vi "Sensor Loop.vi"() -> ()   [LabVIEW 2017]
uses:
  Typedef/FGVAction.ctl
  SimulatorVIs/Simulation Input Global.vi
  <vilib>/ptbypt/NI_PtbyPt.lvlib
panel:
  in  "elevators parameters":T1={"static gain"=10.0, "lag (s)"=0.05, "deadtime (s)"=0.01, "load"=0.0, "deadband"=0.0, "sensor noise"=0.0, "initial PV"=6.0, "plant noise"=0.0} {"plant noise" format="%.2f"; "initial PV" format="%.2f"; "sensor noise" format="%.2f"; "lag (s)" format="%.2f"; "deadtime (s)" format="%.2f"; "deadband" format="%.1f"; "load" format="%.2f"; "static gain" format="%.2f"}
  in  "gripper parameters":T1={"static gain"=2.5, "lag (s)"=2.5, "deadtime (s)"=0.01, "load"=40.0, "deadband"=0.0, "sensor noise"=0.0, "initial PV"=0.0, "plant noise"=0.0} {"plant noise" format="%.2f"; "initial PV" format="%.2f"; "sensor noise" format="%.2f"; "lag (s)" format="%.2f"; "deadtime (s)" format="%.2f"; "deadband" format="%.1f"; "load" format="%.2f"; "static gain" format="%.2f"}
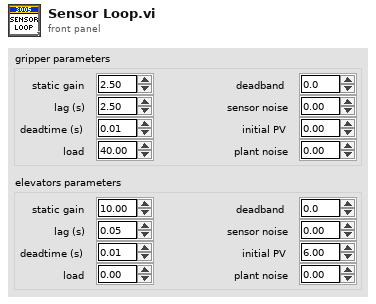
[diagram p1: front panel]
types:
  T1 = cluster{"static gain":dbl, "lag (s)":dbl, "deadtime (s)":dbl, "load":dbl, "deadband":dbl, "sensor noise":dbl, "initial PV":dbl, "plant noise":dbl}
  T2 = typedef "FGVAction.ctl" = enum16{"get", "set"}
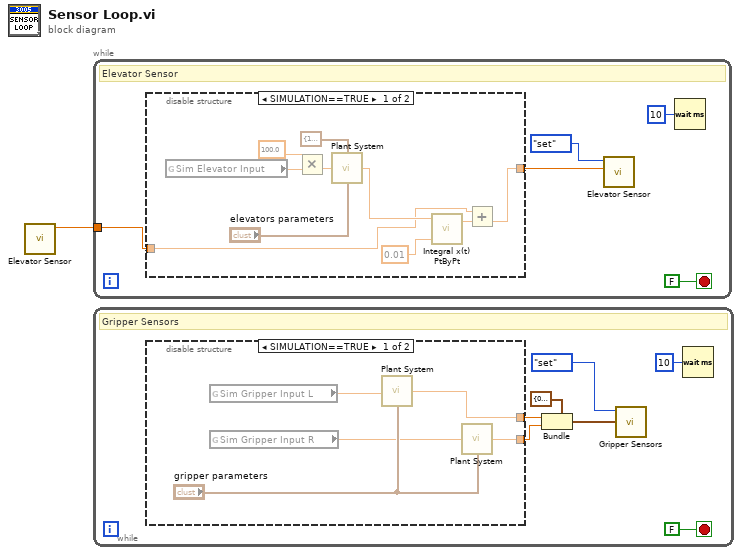
[diagram p0: block diagram]
diagram:
  n1 = call "Elevator Sensor.vi"() -> ("Value"=w1:dbl)  [unwired: 10 in, 1 out]
  n2 = while {
    tunnel: w1 -> [w2]
    stop <- FALSE stop-if-true
    # "Elevator Sensor"
    n3 = disable-structure shown="SIMULATION==TRUE" {
      disable-tunnel: [w8 _] -> w3
      disable-tunnel: w2 -> [w7 _]
      frame condition #0 {
        n4 = global read "Simulation Input Global.vi" "Sim Elevator Input"() -> (w15:dbl)
        n5 = Multiply(x=100.0, y=w15) -> (x*y=w10:dbl)
        n6 = call "Plant System.vi"("output saturation range"=cluster{"output high":dbl, "output low":dbl} {"output high"=100.0, "output low"=-100.0}, "Plant Input"=w10, "process parameters"="elevators parameters") -> ("Plant Output"=w13:dbl)  [unwired: 12 in]
        n7 = call <vilib>:"Integral x(t) PtByPt.vi"("dt"=0.01, "x"=w13) -> ("integral x(t)"=w12:dbl)  [unwired: 2 in, 1 out]
        n8 = Add(x=w7, y=w12) -> (x+y=w8:dbl)
      }
      frame condition #1 (active) {
      }
    }
    n9 = call "Elevator Sensor.vi"("Value"=w3, "Action"=FGVAction."set") -> ()  [unwired: 8 in, 2 out]
    n10 = Wait (ms)(milliseconds to wait=u32 10) -> ()  [unwired: 1 out]
  }
  n11 = while {
    stop <- FALSE stop-if-true
    # "Gripper Sensors"
    n12 = disable-structure shown="SIMULATION==TRUE" {
      disable-tunnel: [w25 _] -> w20
      disable-tunnel: [w24 _] -> w19
      frame condition #0 {
        n13 = global read "Simulation Input Global.vi" "Sim Gripper Input L"() -> (w27:dbl)
        n14 = global read "Simulation Input Global.vi" "Sim Gripper Input R"() -> (w26:dbl)
        n15 = call "Plant System.vi"("Plant Input"=w27, "process parameters"="gripper parameters") -> ("Plant Output"=w25:dbl)  [unwired: 13 in]
        n16 = call "Plant System.vi"("Plant Input"=w26, "process parameters"="gripper parameters") -> ("Plant Output"=w24:dbl)  [unwired: 13 in]
      }
      frame condition #1 (active) {
      }
    }
    n17 = Bundle(cluster=cluster{"Left":dbl, "Right":dbl} {"Left"=0.0, "Right"=0.0} ("Gripper Values"), "Left"=w20, "Right"=w19) -> (w17:cluster{"Left":dbl, "Right":dbl})
    n18 = call "Gripper Sensors.vi"("Input"=w17, "Action"=FGVAction."set") -> ()  [unwired: 8 in, 2 out]
    n19 = Wait (ms)(milliseconds to wait=u32 10) -> ()  [unwired: 1 out]
  }
